vi "Untitled 2 (SubVI).vi"(6 "z 4":dbl[][](array[numeric]), 9 "z 3":dbl[][](array[numeric]), 10 "z 2":dbl[][](array[numeric]), 11 "z":dbl[][](array[numeric])) -> (3 "Array":dbl[][](array[numeric]))   [LabVIEW 2013]
panel:
  out "emptyImageArray":dbl[](array[numeric])
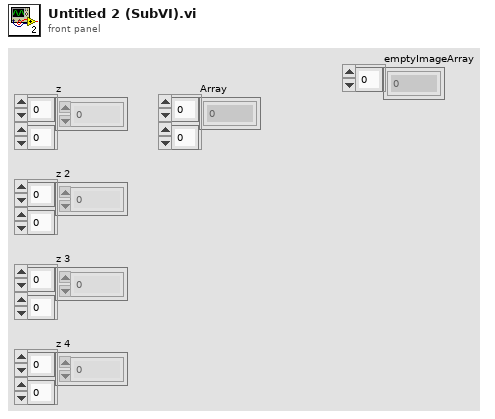
[diagram p1: front panel]
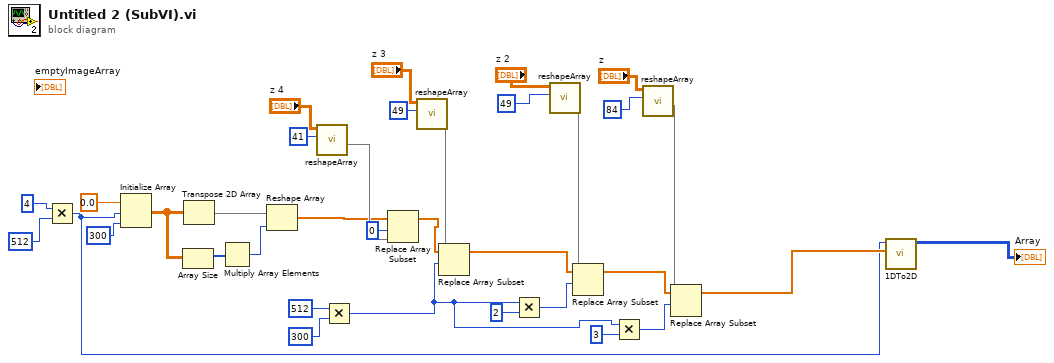
[diagram p0: block diagram]
diagram:
  n1 = Multiply(x=4, y=512) -> (x*y=w14:i32)
  n2 = Initialize Array(0.0, w14, 300 ("dimension size")) -> (w6:dbl[][])
  n3 = Array Size(array=w6) -> (size(s)=w7:i32[])
  n4 = Transpose 2D Array(2D array=w6) -> (transposed array=w5:dbl[][])
  n5 = Multiply Array Elements(1:w7) -> (0:w8:i32)
  n6 = Reshape Array(w5, w8) -> (w9:dbl[])
  n7 = call "reshapeArray.vi"(10:41 ("center"), "z"="z 4") -> (1:w10)  [unwired: 8 in, 1 out]
  n8 = Multiply(x=512, y=300 ("x")) -> (x*y=w28:i32)
  n9 = Replace Array Subset(array=w9, new element=w10, index=0) -> (w17:dbl[])
  n10 = call "reshapeArray.vi"(10:49 ("center"), "z"="z 3") -> (1:w18)  [unwired: 8 in, 1 out]
  n11 = Replace Array Subset(array=w17, new element=w18, index=w28) -> (w21:dbl[])
  n12 = Multiply(x=w28, y=2) -> (x*y=w23:i32)
  n13 = call "reshapeArray.vi"(10:49 ("center"), "z"="z 2") -> (1:w22)  [unwired: 8 in, 1 out]
  n14 = Replace Array Subset(array=w21, new element=w22, index=w23) -> (w25:dbl[])
  n15 = Multiply(x=w28, y=3) -> (x*y=w29:i32)
  n16 = call "reshapeArray.vi"(10:84 ("center"), "z"="z") -> (1:w30)  [unwired: 8 in, 1 out]
  n17 = Replace Array Subset(array=w25, new element=w30, index=w29) -> (w26:dbl[])
  n18 = call "1DTo2D.vi"(10:w26, "reshapeInfo"=w14) -> ("Array out"=→"Array":i16[][])  [unwired: 8 in, 1 out]
